vi "EraseLevelingScans.vi"(11 "Array in":T1[](array[typedef])) -> (3 "All Leveling Scans?":bool)   [LabVIEW 2022 SP3]
uses:
  Controls/ScanParams.ctl
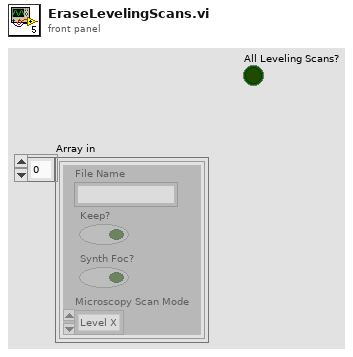
[diagram p1: front panel]
types:
  T1 = typedef "ScanParams.ctl" = cluster{"File Name":string, "Keep?":bool, "Synth Foc?":bool, "Microscopy Scan Mode":enum32{"Level X", "Level Y", "Overview Scan", "Detailed Scan", "V-Z Scan"}}
  T2 = enum32{"Level X", "Level Y", "Overview Scan", "Detailed Scan", "V-Z Scan"}
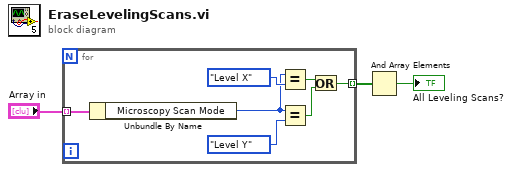
[diagram p0: block diagram]
diagram:
  n1 = for {
    tunnel: "Array in" -> [w10] mode=indexing
    tunnel: [w4] -> w3 mode=indexing
    n2 = Unbundle By Name(w10) -> ("Microscopy Scan Mode"=w7:T2)
    n3 = Equal?(x=w7, y=T2."Level X") -> (x = y?=w6:bool)
    n4 = Equal?(x=w7, y=T2."Level Y") -> (x = y?=w5:bool)
    n5 = Or(x=w6, y=w5) -> (x .or. y?=w4:bool)
  }
  n6 = And Array Elements(Boolean array=w3) -> (logical AND=→"All Leveling Scans?":bool)
